vi "FGen FGV.vi"(7 "Action":T2, 8 "error in (no error)":errorcluster, 11 "FGen":T1) -> (0 "error out":errorcluster, 3 "FGen Out":T1)   [LabVIEW 2021]
uses:
  Controls/FGen FGV Enum.ctl
  Controls/FGen Desktop Configuration.ctl
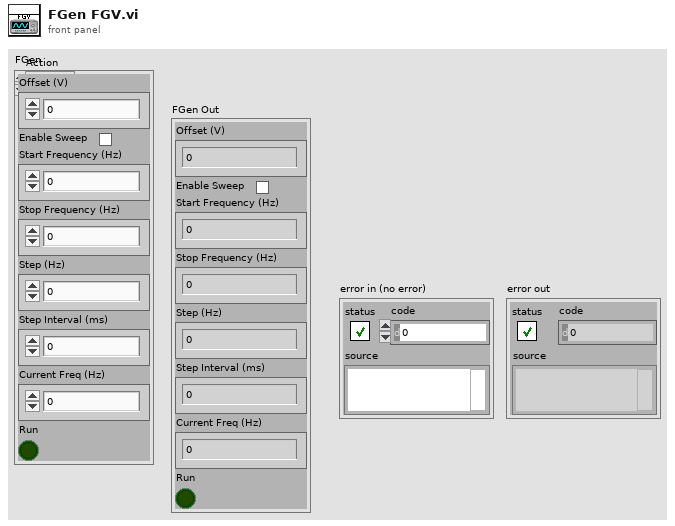
[diagram p1: front panel]
types:
  T1 = typedef "FGen Desktop Configuration.ctl" = cluster{"Offset (V)":dbl, "Enable Sweep":bool, "Start Frequency (Hz)":dbl, "Stop Frequency (Hz)":dbl, "Step (Hz)":dbl, "Step Interval (ms)":dbl, "Current Freq (Hz)":dbl, "Run":bool}
  T2 = typedef "FGen FGV Enum.ctl" = enum16{"Set", "Get"}
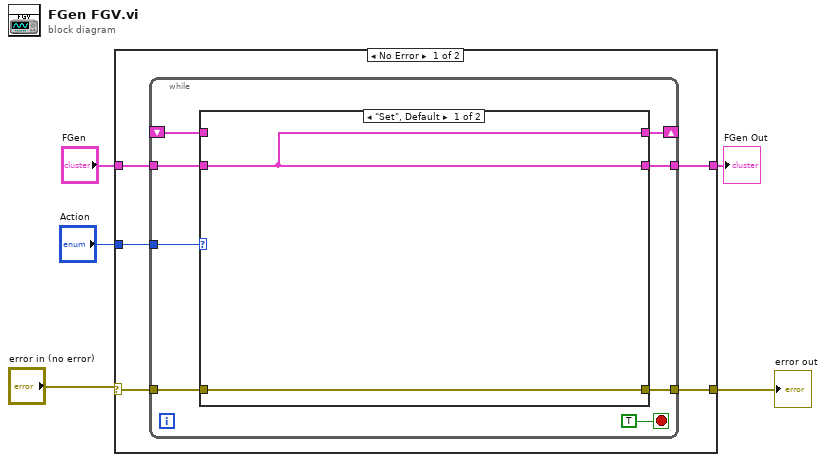
[diagram p0: block diagram]
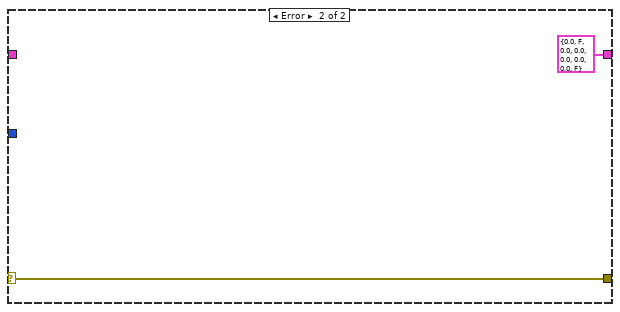
[diagram p3: hidden frame]
diagram:
  n1 = case shown="No Error" "error in (no error)" {
    selector: "error in (no error)" -> [w8 w24]
    tunnel: "Action" -> [w10 _]
    tunnel: "FGen" -> [w9 _]
    tunnel: [w7 w24] -> w2
    tunnel: [w6 T1 {"Offset (V)"=0.0, "Enable Sweep"=FALSE, "Start Frequency (Hz)"=0.0, "Stop Frequency (Hz)"=0.0, "Step (Hz)"=0.0, "Step Interval (ms)"=0.0, "Current Freq (Hz)"=0.0, "Run"=FALSE} ("FGen")] -> w1
    frame No Error {
      n2 = while {
        tunnel: w10 -> [w17]
        tunnel: w9 -> [w16]
        shift-right: [w15] -> _
        shift-left: _ -> [w14]
        tunnel: [w13] -> w6
        tunnel: w8 -> [w12]
        tunnel: [w11] -> w7
        stop <- TRUE stop-if-true
        n3 = case shown="\"Set\", Default" w17 {
          tunnel: w16 -> [w19 _]
          tunnel: [w19 w22] -> w15
          tunnel: w14 -> [_ w22]
          tunnel: [w19 w22] -> w13
          tunnel: w12 -> [w20 w21]
          tunnel: [w20 w21] -> w11
          frame "Set", Default {
          }
          frame "Get" {
          }
        }
      }
    }
    frame Error {
    }
  }
  "error out" <- w2
  "FGen Out" <- w1
